vi "AuMT8852B EDR Sensitivity Results LEG.vi"(8 "error in (no error)":errorcluster, 11 "VISA session":refnum<visa-resource-name>) -> (0 "error out":errorcluster, 2 "error code":i32, 3 "VISA session out":refnum<visa-resource-name>, 4 "Results":T1 {"Overall BER" format="%.2e"; "Overall BER" format="%.2e"})   [LabVIEW 2017]
doc: "Anritsu MT8852B Bluetooth Tester\n\n<B>NOTE:</B> USE THIS VI ONLY FOR MT8852B FIRMWARE VERSIONS UP TO AND INCLUDING 4.08.100\n\nReturns the summary results of the EDR Sensitivity test.\n\nOUTPUT\nResults - measurements made during the test."
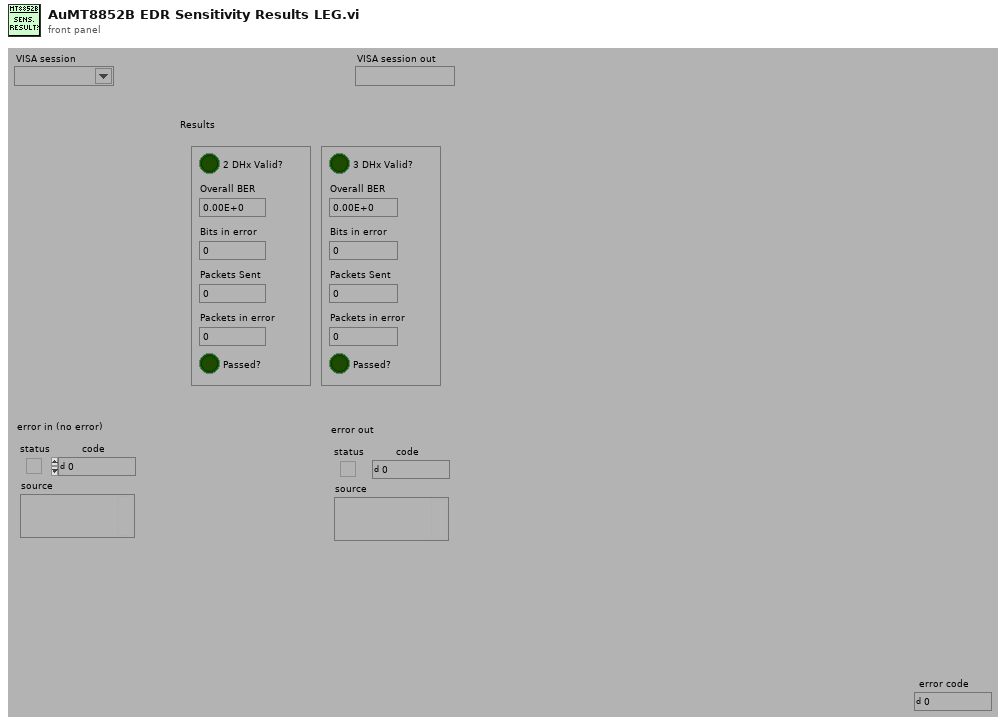
[diagram p1: front panel]
types:
  T1 = cluster{"2 DHx Valid?":bool, "Overall BER":dbl, "Bits in error":u32, "Packets Sent":u32, "Passed?":bool, "Packets in error":u32, "3 DHx Valid?":bool, "Overall BER":dbl, "Bits in error":u32, "Packets Sent":u32, "Passed?":bool, "Packets in error":u32}
  T2 = enum16{"Simulate", "Range check", "Cache", "Query instrument status"}
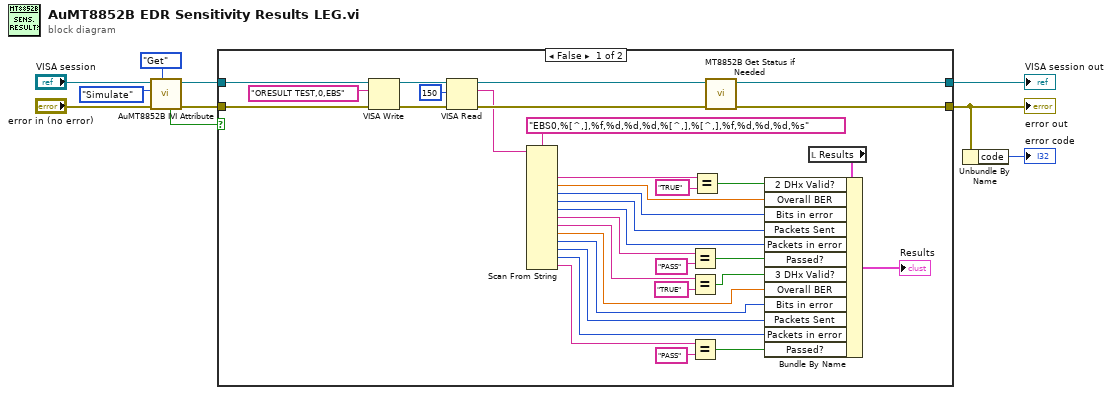
[diagram p0: block diagram]
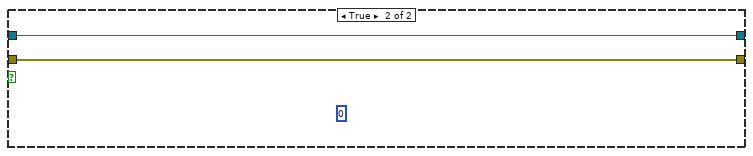
[diagram p2: hidden frame]
diagram:
  n1 = call <instrlib>:"AuMT8852B IVI Attribute.vi"("Set/Get (Set)"=enum16{"Set", "Get"}."Get", "error in (no error)"="error in (no error)", "Flag (Simulate)"=T2."Simulate", "VISA session"="VISA session") -> ("error out"=w7:errorcluster, "VISA session out"=w9:refnum<visa-resource-name>, "Value out"=w3:bool)  [unwired: 5 in]
  n2 = case shown="False" w3 {
    tunnel: [w36 w46] -> w10
    tunnel: [w35 w45] -> w1
    tunnel: w9 -> [w43 w46]
    tunnel: w7 -> [w42 w45]
    frame False {
      n3 = VISA Write(VISA resource name=w43, write buffer="ORESULT TEST,0,EBS" ("write buffer (\"\")"), error in (no error)=w42) -> (VISA resource name out=w41:refnum<visa-resource-name>, error out=w40:errorcluster)  [unwired: 1 out]
      n4 = VISA Read(VISA resource name=w41, byte count=u32 150 ("byte count (0)"), error in (no error)=w40) -> (VISA resource name out=w34:refnum<visa-resource-name>, read buffer=w32:string, error out=w33:errorcluster)  [unwired: 1 out]
      n5 = Scan From String(format string="EBS0,%[^,],%f,%d,%d,%d,%[^,],%[^,],%f,%d,%d,%d,%s" ("Format String"), input string=w32) -> (output 1=w31:string, output 2=w27:dbl, output 3=w26:i32, output 4=w25:i32, output 5=w23:i32, output 6=w22:string, output 7=w18:string, output 8=w17:dbl, output 9=w16:i32, output 10=w15:i32, output 11=w14:i32, output 12=w13:string)  [unwired: 14 in, 3 out]
      n6 = Equal?(x=w22, y="PASS") -> (x = y?=w21:bool)
      n7 = Equal?(x=w18, y="TRUE") -> (x = y?=w19:bool)
      n8 = Equal?(x=w13, y="PASS") -> (x = y?=w12:bool)
      n9 = Equal?(x=w31, y="TRUE") -> (x = y?=w28:bool)
      n10 = call <instrlib>:"MT8852B Get Status if Needed.vi"("error in (no error)"=w33, "VISA session"=w34) -> ("error out"=w35:errorcluster, "VISA session out"=w36:refnum<visa-resource-name>)  [unwired: 8 in]
      n11 = local read "Results"() -> (w29:T1)
      n12 = Bundle By Name(cluster=w29, "2 DHx Valid?"=w28, "Overall BER"=w27, "Bits in error"=w26, "Packets Sent"=w25, "Packets in error"=w23, "Passed?"=w21, "3 DHx Valid?"=w19, "Overall BER"=w17, "Bits in error"=w16, "Packets Sent"=w15, "Packets in error"=w14, "Passed?"=w12) -> (→"Results":T1)
    }
    frame True {
      (unwired) u8 0
    }
  }
  "error out" <- w1
  "VISA session out" <- w10
  n13 = Unbundle By Name(w1) -> ("code"=→"error code":i32)
